vi "Construct TCP Server.vi"(9 "Port":u16, 10 "Net Address":u32, 11 "Service Name":string) -> (3 "TCP Server out":refnum<class "TCP Server.lvclass">)   [LabVIEW 2019, in "TCP Interface.lvlib" / "TCP Server.lvclass"]
uses:
  <vilib>/gpm_packages/@cs/Network-Sink/Source/TCP Interface/TCP Server/TCP Server.lvclass
  <vilib>/gpm_packages/@cs/Network-Sink/Source/TCP Interface/TCP Server/TCP Server.lvclass/TCP Server.ctl
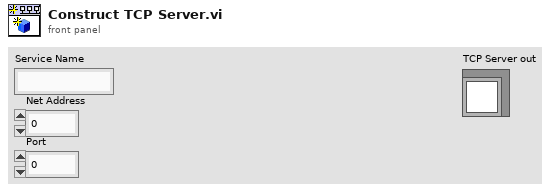
[diagram p1: front panel]
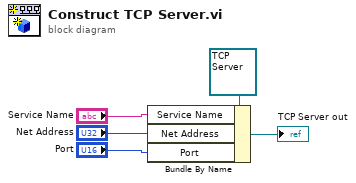
[diagram p0: block diagram]
diagram:
  n1 = Bundle By Name(cluster=refnum<class "TCP Server.lvclass"> refnum ("TCP Server in"), "Service Name"="Service Name", "Net Address"="Net Address", "Port"="Port") -> (→"TCP Server out":refnum<class "TCP Server.lvclass">)
